vi "test6-ChainNodeExitSequenceCheck.vi"(8 "error in (no error)":errorcluster, 11 "TestCase in":refnum<class "testcase-CSMChainMode.lvclass">) -> (0 "error out":errorcluster, 3 "TestCase out":refnum<class "testcase-CSMChainMode.lvclass">)   [LabVIEW 2017, in "testcase-CSMChainMode.lvclass"]
uses:
  testcase-CSMChainMode.lvclass
  <vilib>/addons/_JKI Toolkits/VI Tester/TestCase.llb/TestCase.lvclass
  src/user.lib/_NEVSTOP/Communicable State Machine(CSM)/Communicable State Machine.lvlib
  C:/Program Files (x86)/National Instruments/LabVIEW 2017/vi.lib/addons/_JKI Toolkits/VI Tester/TestCase.llb/TestCase.lvclass
panel:
  out "Loop Count":i32
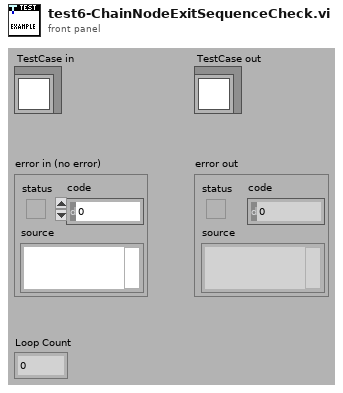
[diagram p1: front panel]
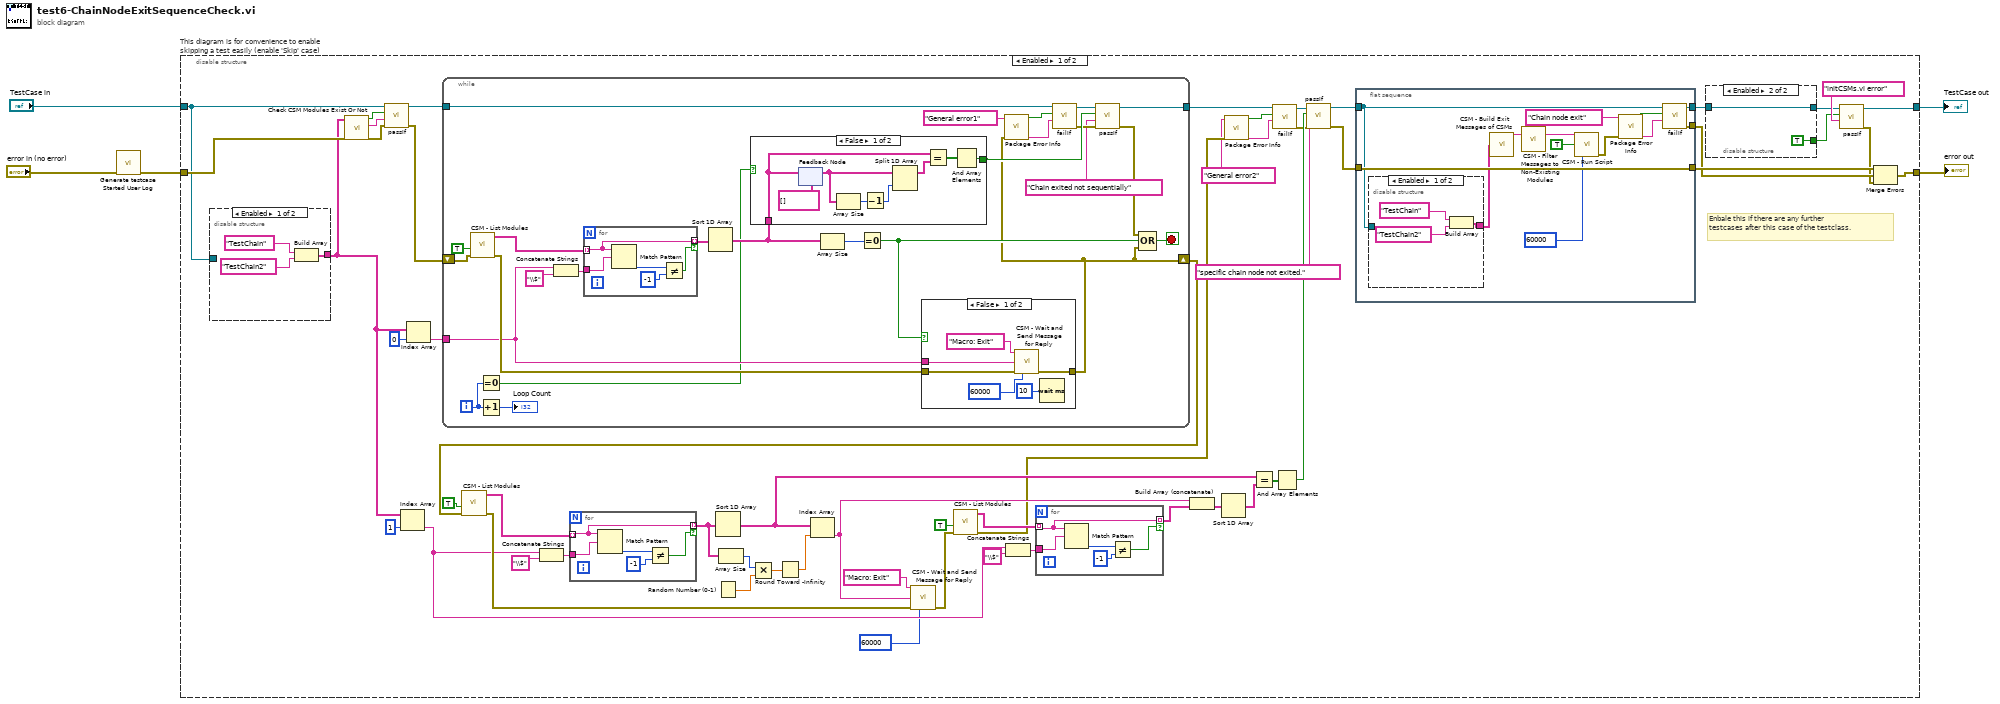
[diagram p0: block diagram]
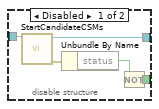
[diagram p2: hidden frame]
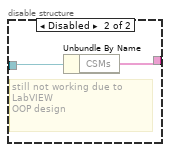
[diagram p3: hidden frame]
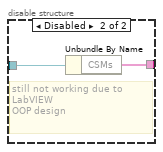
[diagram p4: hidden frame]
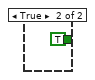
[diagram p6: hidden frame]
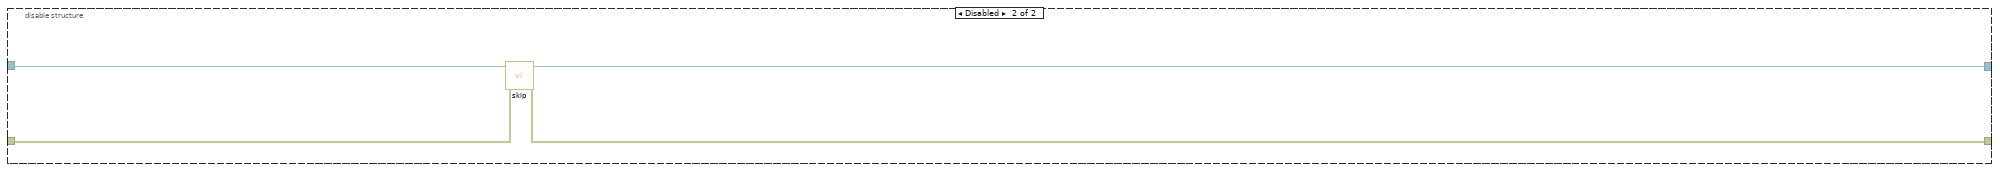
[diagram p7: hidden frame]
diagram:
  n1 = call "Generate testcase Started User Log.vi"("Error In"="error in (no error)") -> ("error out"=w1:errorcluster)  [unwired: 10 in]
  n2 = disable-structure "This diagram is for convenience to enable skipping a test easily (enable 'Skip' case)" shown="Enabled" {
    disable-tunnel: "TestCase in" -> [w7 w152]
    disable-tunnel: [w13 w150] -> w2
    disable-tunnel: [w12 w151] -> w4
    disable-tunnel: w1 -> [w27 w149]
    frame Enabled {
      # "Enbale this if there are any further\ntestcases after this case of the testclass."
      n3 = disable-structure shown="Enabled" {
        disable-tunnel: [w69 w72] -> w8
        disable-tunnel: w7 -> [_ w73]
        frame Enabled {
          n4 = Build Array("TestChain" ("CSM Name"), "TestChain2" ("CSM Name")) -> (w69:string[])
        }
        frame Disabled {
          # "still not working due to \nLabVIEW\nOOP design"
          n5 = Unbundle By Name(w73) -> ("CSMs"=w72:string[])
        }
      }
      n6 = call "Check CSM Modules Exist Or Not.vi"("error in"=w27, "CSM names in"=w8) -> ("error out"=w29:errorcluster, "Debug string"=w30:string, "All Modules Exist?"=w31:bool)  [unwired: 7 in]
      n7 = call-dynamic "passIf.vi"("error in (no error)"=w29, "message (\"\")"=w30, "pass"=w31, "TestCase in"=w7) -> ("error out"=w26:errorcluster, "TestCase out"=w28:refnum<class "testcase-CSMChainMode.lvclass">)  [unwired: 6 in]
      n8 = Index Array(array=w8, index=1) -> (element=w42:string)
      n9 = Index Array(array=w8, index=0) -> (element=w60:string)
      n10 = while {
        tunnel: w60 -> [w121]
        tunnel: w28 -> [w108]
        tunnel: [w120] -> w22
        shift-right: [w104] -> w25
        shift-left: w26 -> [w117]
        i -> [w115]
        stop <- w119 stop-if-true
        n11 = call "CSM - List Modules.vi"("Error In"=w117, "With Nodes? (F)"=TRUE) -> ("error out"=w122:errorcluster, "Module Names"=w124:string[])  [unwired: 8 in]
        n12 = Equal To 0?(x=w115) -> (x = 0?=w112:bool)
        n13 = Increment(x=w115) -> (x+1=→"Loop Count":i32)
        n14 = Concatenate Strings(w121, "\\$" ("string")) -> (w127:string)
        n15 = for {
          tunnel: w124 -> [w146] mode=indexing
          tunnel: [w146] -> w116 mode=indexing if=w145
          tunnel: w127 -> [w144]
          n16 = Match Pattern(string=w146, regular expression=w144) -> (offset past match=w148:i32)  [unwired: 1 in, 3 out]
          n17 = Not Equal?(x=w148, y=-1) -> (x != y?=w145:bool)
        }
        n18 = Sort 1D Array(array=w116) -> (sorted array=w114:string[])
        n19 = case shown="False" w112 {
          tunnel: w114 -> [w138 _]
          tunnel: [w135 TRUE] -> w113
          frame False {
            n20 = feedback #1(string[] []) -> (w141:string[])
            n21 = feedback-in #1(w138) -> ()
            n22 = Array Size(array=w141) -> (size(s)=w140:i32)
            n23 = Decrement(x=w140) -> (x-1=w139:i32)
            n24 = Split 1D Array(array=w141, index=w139) -> (first subarray=w137:string[])  [unwired: 1 out]
            n25 = Equal?(x=w138, y=w137) -> (x = y?=w136:bool[])
            n26 = And Array Elements(Boolean array=w136) -> (logical AND=w135:bool)
          }
          frame True {
          }
        }
        n27 = Array Size(array=w114) -> (size(s)=w123:i32)
        n28 = Equal To 0?(x=w123) -> (x = 0?=w111:bool)
        n29 = case shown="False" w111 {
          tunnel: w122 -> [w133 w134]
          tunnel: w121 -> [w132 _]
          tunnel: [w130 w134] -> w104
          frame False {
            n30 = call "CSM - Wait and Send Message for Reply.vi"("State"="Macro: Exit", "Target Module"=w132, "Error In (No Error)"=w133, "Response Timeout (-2 Using Global Settings)"=60000) -> ("error out"=w130:errorcluster)  [unwired: 8 in, 3 out]
            n31 = Wait (ms)(milliseconds to wait=u32 10) -> ()  [unwired: 1 out]
          }
          frame True {
          }
        }
        n32 = call "Package Error Info.vi"("error in"=w104, "String in"="General error1") -> ("packed error info out"=w109:string, "error status"=w110:bool)  [unwired: 8 in]
        n33 = call-dynamic "failIf.vi"("message (\"\")"=w109, "fail"=w110, "TestCase in"=w108) -> ("error out"=w106:errorcluster, "TestCase out"=w107:refnum<class "testcase-CSMChainMode.lvclass">)  [unwired: 7 in]
        n34 = call-dynamic "passIf.vi"("error in (no error)"=w106, "message (\"\")"="Chain exited not sequentially" ("message (\"\")"), "pass"=w113, "TestCase in"=w107) -> ("error out"=w105:errorcluster, "TestCase out"=w120:refnum<class "testcase-CSMChainMode.lvclass">)  [unwired: 6 in]
        n35 = Compound Arithmetic op=OR(w105, w111, w104) -> (w119:bool)
      }
      n36 = call "CSM - List Modules.vi"("Error In"=w25, "With Nodes? (F)"=TRUE) -> ("error out"=w48:errorcluster, "Module Names"=w58:string[])  [unwired: 8 in]
      n37 = Concatenate Strings(w42, "\\$" ("string")) -> (w55:string)
      n38 = for {
        tunnel: w58 -> [w99] mode=indexing
        tunnel: [w99] -> w54 mode=indexing if=w98
        tunnel: w55 -> [w97]
        n39 = Match Pattern(string=w99, regular expression=w97) -> (offset past match=w101:i32)  [unwired: 1 in, 3 out]
        n40 = Not Equal?(x=w101, y=-1) -> (x != y?=w98:bool)
      }
      n41 = Sort 1D Array(array=w54) -> (sorted array=w37:string[])
      n42 = Random Number (0-1)() -> (number: 0 to 1=w52:dbl)
      n43 = Array Size(array=w54) -> (size(s)=w53:i32)
      n44 = Multiply(x=w53, y=w52) -> (x*y=w51:dbl)
      n45 = Round Toward -Infinity(1:w51) -> (0:w50:dbl)
      n46 = Index Array(array=w37, index=w50) -> (element=w40:string)
      n47 = call "CSM - Wait and Send Message for Reply.vi"("State"="Macro: Exit", "Target Module"=w40, "Error In (No Error)"=w48, "Response Timeout (-2 Using Global Settings)"=60000) -> ("error out"=w44:errorcluster)  [unwired: 8 in, 3 out]
      n48 = call "CSM - List Modules.vi"("Error In"=w44, "With Nodes? (F)"=TRUE) -> ("error out"=w19:errorcluster, "Module Names"=w43:string[])  [unwired: 8 in]
      n49 = Concatenate Strings(w42, "\\$" ("string")) -> (w47:string)
      n50 = for {
        tunnel: [w92] -> w41 mode=indexing if=w94
        tunnel: w47 -> [w93]
        tunnel: w43 -> [w92] mode=indexing
        n51 = Match Pattern(string=w92, regular expression=w93) -> (offset past match=w96:i32)  [unwired: 1 in, 3 out]
        n52 = Not Equal?(x=w96, y=-1) -> (x != y?=w94:bool)
      }
      n53 = Build Array (concatenate)(w40, w41) -> (w39:string[])
      n54 = Sort 1D Array(array=w39) -> (sorted array=w38:string[])
      n55 = call "Package Error Info.vi"("error in"=w19, "String in"="General error2") -> ("packed error info out"=w24:string, "error status"=w23:bool)  [unwired: 8 in]
      n56 = Equal?(x=w37, y=w38) -> (x = y?=w36:bool[])
      n57 = call-dynamic "failIf.vi"("message (\"\")"=w24, "fail"=w23, "TestCase in"=w22) -> ("error out"=w20:errorcluster, "TestCase out"=w21:refnum<class "testcase-CSMChainMode.lvclass">)  [unwired: 7 in]
      n58 = And Array Elements(Boolean array=w36) -> (logical AND=w35:bool)
      n59 = call-dynamic "passIf.vi"("error in (no error)"=w20, "message (\"\")"="specific chain node not exited.", "pass"=w35, "TestCase in"=w21) -> ("error out"=w32:errorcluster, "TestCase out"=w34:refnum<class "testcase-CSMChainMode.lvclass">)  [unwired: 6 in]
      n60 = flat-sequence {
        tunnel: w34 -> [w75]
        tunnel: [w80] -> w33
        tunnel: w32 -> [w83]
        tunnel: [w83] -> w11
        tunnel: [w77] -> w10
        frame #0 {
          n61 = disable-structure shown="Enabled" {
            disable-tunnel: [w87 w90] -> w76
            disable-tunnel: w75 -> [_ w91]
            frame Enabled {
              n62 = Build Array("TestChain" ("CSM Name"), "TestChain2" ("CSM Name")) -> (w87:string[])
            }
            frame Disabled {
              # "still not working due to \nLabVIEW\nOOP design"
              n63 = Unbundle By Name(w91) -> ("CSMs"=w90:string[])
            }
          }
          n64 = call "CSM - Build Exit Messages of CSMs.vi"("CSMs"=w76) -> ("States"=w85:string)  [unwired: 14 in]
          n65 = call "CSM - Filter Messages to Non-Existing Modules.vi"("States In"=w85) -> ("States Out"=w86:string)  [unwired: 14 in]
          n66 = call "CSM - Run Script.vi"("CSM Scripts"=w86, "Continue If Error? (F)"=TRUE, "Response Timeout (-2 Using Global Settings)"=60000) -> ("error out"=w79:errorcluster)  [unwired: 10 in, 2 out]
          n67 = call "Package Error Info.vi"("error in"=w79, "String in"="Chain node exit") -> ("packed error info out"=w82:string, "error status"=w81:bool)  [unwired: 8 in]
          n68 = call-dynamic "failIf.vi"("message (\"\")"=w82, "fail"=w81, "TestCase in"=w75) -> ("error out"=w77:errorcluster, "TestCase out"=w80:refnum<class "testcase-CSMChainMode.lvclass">)  [unwired: 7 in]
        }
      }
      n69 = disable-structure shown="Enabled" {
        disable-tunnel: w33 -> [w66 w68]
        disable-tunnel: [w65 TRUE ("pass")] -> w15
        disable-tunnel: [w64 w68] -> w14
        frame Disabled {
          n70 = call "StartCandidateCSMs.vi"("TestCase in"=w66) -> ("error out"=w63:errorcluster, "TestCase out"=w64:refnum<class "testcase-CSMChainMode.lvclass">)  [unwired: 9 in]
          n71 = Unbundle By Name(w63) -> ("status"=w62:bool)
          n72 = Not(x=w62) -> (.not. x?=w65:bool)
        }
        frame Enabled {
        }
      }
      n73 = call-dynamic "passIf.vi"("message (\"\")"="initCSMs.vi error" ("message (\"\")"), "pass"=w15, "TestCase in"=w14) -> ("error out"=w9:errorcluster, "TestCase out"=w13:refnum<class "testcase-CSMChainMode.lvclass">)  [unwired: 7 in]
      n74 = Merge Errors(w11, w10, w9) -> (w12:errorcluster)
    }
    frame Disabled {
      # "skip test result while test is under development"
      n75 = call <vilib>:"skip.vi"("error in (no error)"=w149, "TestCase in"=w152) -> ("error out"=w151:errorcluster, "TestCase out"=w150:refnum<class "testcase-CSMChainMode.lvclass">)  [unwired: 8 in]
    }
  }
  "error out" <- w4
  "TestCase out" <- w2
